vi "SensorColorSubVI.vi"(6 "Frecuencia in":bool, 7 "Frecuencia 1":bool=TRUE) -> (0 "Rojo":dbl format="%.2f", 1 "Azul":dbl, 2 "Verde":dbl format="%.2f", 3 "Sin Filtro":dbl format="%.2f")   [LabVIEW 2017]
uses:
  enumColor.ctl
  <vilib>/DAQmx/write.llb/DAQmx Write (Digital 1D Bool 1Chan 1Samp).vi
  <vilib>/DAQmx/read.llb/DAQmx Read (Counter DBL 1Chan 1Samp).vi
  <vilib>/DAQmx/create/channels.llb/DAQmx Create Channel (DO-Digital Output).vi
  <vilib>/DAQmx/create/channels.llb/DAQmx Create Channel (CI-Count Edges).vi
  <vilib>/DAQmx/miscellaneous.llb/DAQmx Fill In Error Info.vi
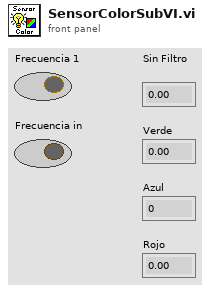
[diagram p1: front panel]
types:
  T1 = typedef "enumColor.ctl" = enum16{"Inicio", "SinFiltro1", "SinFiltro2", "SinFiltro3", "Rojo1", "Rojo2", "Rojo3", "Verde1", "Verde2", "Verde3", "Azul1", "Azul2", "Azul3", "Cierre"}
  T2 = cluster{"task out":refnum<k21>, "error out":errorcluster}
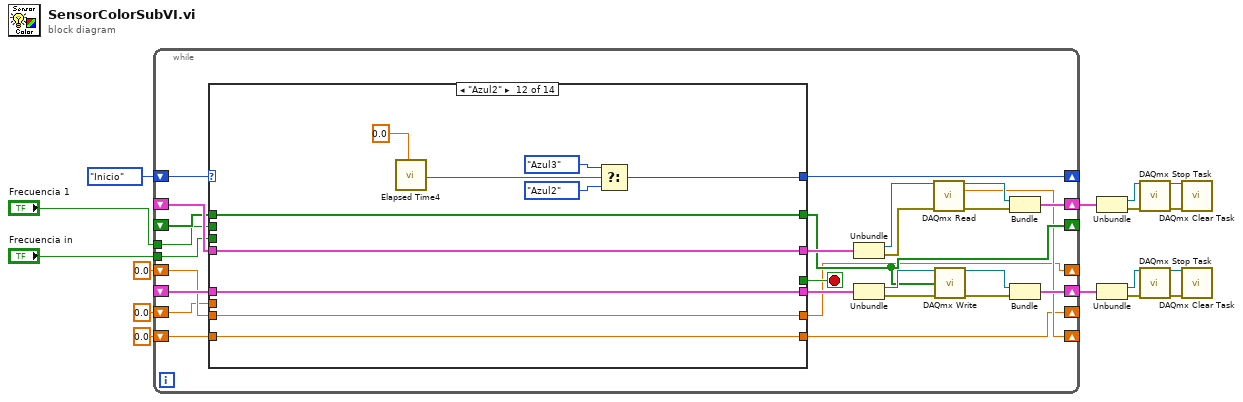
[diagram p0: block diagram]
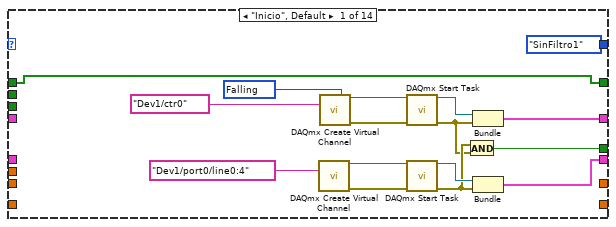
[diagram p2: hidden frame]
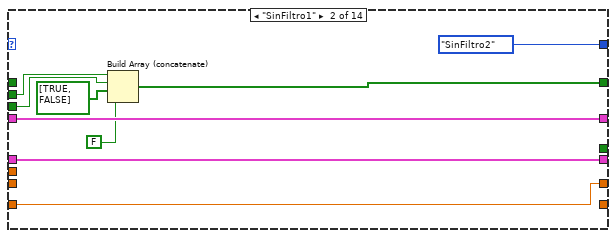
[diagram p3: hidden frame]
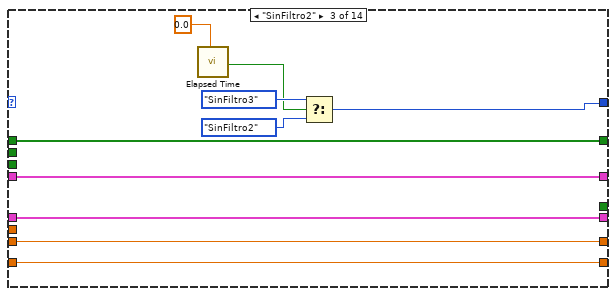
[diagram p4: hidden frame]
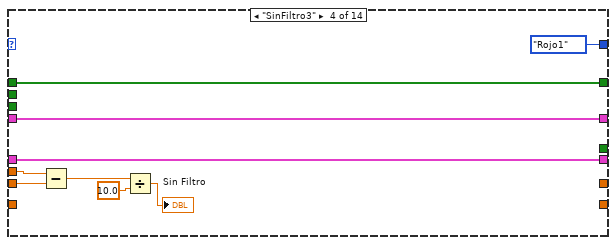
[diagram p5: hidden frame]
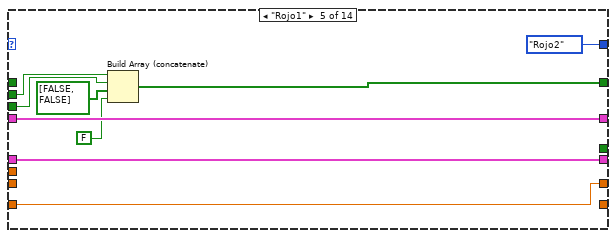
[diagram p6: hidden frame]
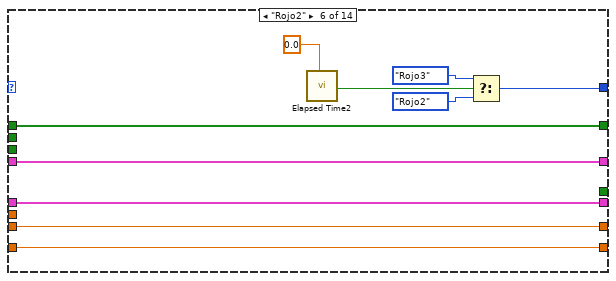
[diagram p7: hidden frame]
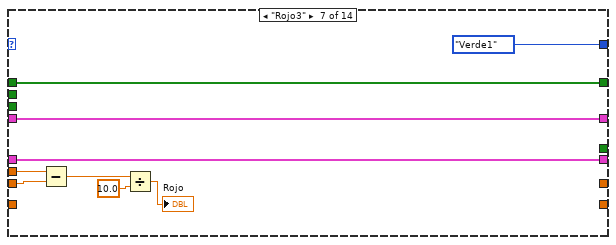
[diagram p8: hidden frame]
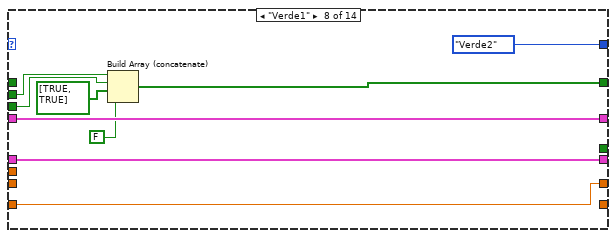
[diagram p9: hidden frame]
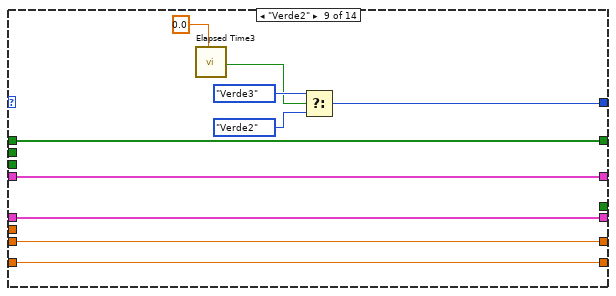
[diagram p10: hidden frame]
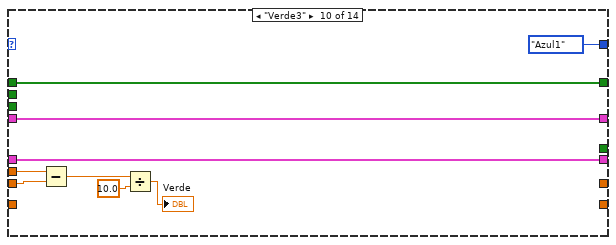
[diagram p11: hidden frame]
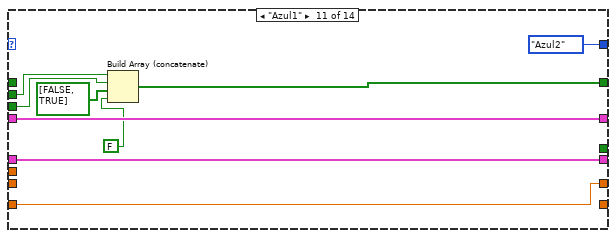
[diagram p12: hidden frame]
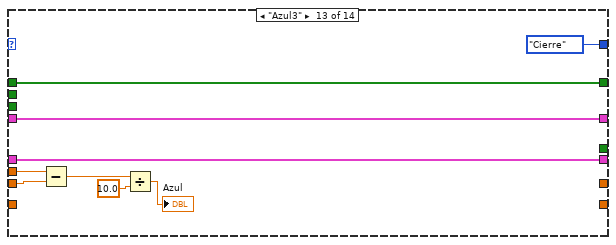
[diagram p13: hidden frame]
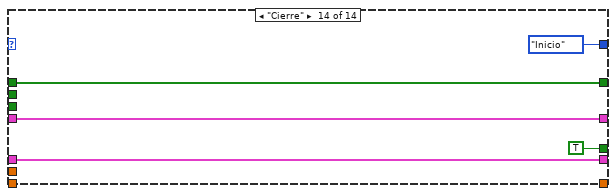
[diagram p14: hidden frame]
diagram:
  n1 = while {
    shift-right: [w42] -> _
    shift-left: enumColor."Inicio" -> [w27]
    shift-right: [w28] -> w14
    shift-left: _ -> [w29]
    shift-right: [w36] -> w13
    shift-left: _ -> [w33]
    tunnel: "Frecuencia 1" -> [w17]
    tunnel: "Frecuencia in" -> [w18]
    shift-right: [w26] -> _
    shift-left: _ -> [w25]
    shift-right: [w24] -> _
    shift-left: 0.0 ("data") -> [w23]
    shift-right: [w22] -> _
    shift-left: 0.0 ("data") -> [w21]
    shift-right: [w20] -> _
    shift-left: 0.0 ("data") -> [w19]
    stop <- w43 stop-if-true
    n2 = case shown="\"Azul2\"" w27 {
      tunnel: [w55 _ _ _ _ _ _ _ _ _ _ _ _ TRUE] -> w43
      tunnel: [w49 w68 w78 w87 w92 w106 w114 w119 w134 w142 w147 w162 w170 w175] -> w39
      tunnel: [enumColor."SinFiltro1" enumColor."SinFiltro2" w70 enumColor."Rojo1" enumColor."Rojo2" w102 enumColor."Verde1" enumColor."Verde2" w130 enumColor."Azul1" enumColor."Azul2" w158 enumColor."Cierre" enumColor."Inicio"] -> w42
      tunnel: w17 -> [_ w65 _ _ w95 _ _ w123 _ _ w151 _ _ _]
      tunnel: w18 -> [_ w64 _ _ w94 _ _ w122 _ _ w150 _ _ _]
      tunnel: [w46 w63 w77 w86 w93 w101 w113 w121 w129 w141 w149 w157 w169 w172] -> w26
      tunnel: w33 -> [_ w68 w78 w87 w92 w106 w114 w119 w134 w142 w147 w162 w170 w175]
      tunnel: [w47 w67 w76 w85 w91 w105 w115 w120 w133 w143 w148 w161 w171 w176] -> w30
      tunnel: w29 -> [_ w67 w76 w85 w91 w105 w115 w120 w133 w143 w148 w161 w171 w176]
      tunnel: w25 -> [w46 _ w77 w86 _ w101 w113 _ w129 w141 _ w157 w169 w172]
      tunnel: w23 -> [_ w61 w71 _ w89 w98 _ w117 w126 _ w146 w155 _ _]
      tunnel: [_ w61 w72 _ w89 w99 _ w117 w128 _ w146 w156 _ _] -> w22
      tunnel: w21 -> [_ _ w72 w80 _ w99 w112 _ w128 w139 _ w156 w165 _]
      tunnel: [_ _ w71 _ _ w98 _ _ w126 _ _ w155 _ _] -> w20
      tunnel: w19 -> [_ _ _ w81 _ _ w111 _ _ w140 _ _ w166 _]
      frame "Inicio", Default {
        w44 = 10171 items=["Rising"=10280, "Falling"=10171] ("edge")
        n3 = call-poly <vilib>:"DAQmx Create Virtual Channel.vi"("lines"=tag "Dev1/port0/line0:4") -> ("task out"=w59:refnum<k21>, "error out"=w58:errorcluster)  [unwired: 13 in]
        n4 = call-poly <vilib>:"DAQmx Create Virtual Channel.vi"("edge"=w44, "counter"=tag "Dev1/ctr0") -> ("task out"=w57:refnum<k21>, "error out"=w56:errorcluster)  [unwired: 12 in]
        n5 = call <vilib>:"DAQmx Start Task.vi"("task/channels in"=w57, "error in"=w56) -> ("task out"=w51:refnum<k21>, "error out"=w50:errorcluster)  [unwired: 12 in]
        n6 = call <vilib>:"DAQmx Start Task.vi"("task/channels in"=w59, "error in"=w58) -> ("task out"=w53:refnum<k21>, "error out"=w52:errorcluster)  [unwired: 12 in]
        n7 = And(x=w52, y=w50) -> (x .and. y?=w55:bool)
        n8 = Bundle("task out"=w51, "error out"=w50) -> (w49:T2)  [unwired: 1 in]
        n9 = Bundle("task out"=w53, "error out"=w52) -> (w47:T2)  [unwired: 1 in]
      }
      frame "SinFiltro1" {
        n10 = Build Array (concatenate)(w65, w64, bool[] [TRUE, FALSE], FALSE) -> (w63:bool[])
      }
      frame "SinFiltro2" {
        n11 = call "Elapsed Time"("Set Start Time (s)"=0.0) -> ("Time has Elapsed"=w73:bool)  [unwired: 11 in, 7 out]
        n12 = Select(t=enumColor."SinFiltro3", s=w73, f=enumColor."SinFiltro2") -> (s? t:f=w70:T1)
      }
      frame "SinFiltro3" {
        n13 = Subtract(x=w81, y=w80) -> (x-y=w84:dbl)
        n14 = Divide(x=w84, y=10.0) -> (x/y=→"Sin Filtro":dbl)
      }
      frame "Rojo1" {
        n15 = Build Array (concatenate)(w95, w94, bool[] [FALSE, FALSE], FALSE) -> (w93:bool[])
      }
      frame "Rojo2" {
        n16 = call "Elapsed Time2"("Set Start Time (s)"=0.0) -> ("Time has Elapsed"=w100:bool)  [unwired: 11 in, 7 out]
        n17 = Select(t=enumColor."Rojo3", s=w100, f=enumColor."Rojo2") -> (s? t:f=w102:T1)
      }
      frame "Rojo3" {
        n18 = Subtract(x=w111, y=w112) -> (x-y=w110:dbl)
        n19 = Divide(x=w110, y=10.0) -> (x/y=→"Rojo":dbl)
      }
      frame "Verde1" {
        n20 = Build Array (concatenate)(w123, w122, bool[] [TRUE, TRUE], FALSE) -> (w121:bool[])
      }
      frame "Verde2" {
        n21 = call "Elapsed Time3"("Set Start Time (s)"=0.0) -> ("Time has Elapsed"=w127:bool)  [unwired: 11 in, 7 out]
        n22 = Select(t=enumColor."Verde3", s=w127, f=enumColor."Verde2") -> (s? t:f=w130:T1)
      }
      frame "Verde3" {
        n23 = Subtract(x=w140, y=w139) -> (x-y=w137:dbl)
        n24 = Divide(x=w137, y=10.0 ("x")) -> (x/y=→"Verde":dbl)
      }
      frame "Azul1" {
        n25 = Build Array (concatenate)(w151, w150, bool[] [FALSE, TRUE], FALSE) -> (w149:bool[])
      }
      frame "Azul2" {
        n26 = call "Elapsed Time4"("Set Start Time (s)"=0.0) -> ("Time has Elapsed"=w154:bool)  [unwired: 11 in, 7 out]
        n27 = Select(t=enumColor."Azul3", s=w154, f=enumColor."Azul2") -> (s? t:f=w158:T1)
      }
      frame "Azul3" {
        n28 = Subtract(x=w166, y=w165) -> (x-y=w167:dbl)
        n29 = Divide(x=w167, y=10.0) -> (x/y=→"Azul":dbl)
      }
      frame "Cierre" {
      }
    }
    n30 = Unbundle(w39) -> ("task out"=w38:refnum<k21>, "error out"=w37:errorcluster)
    n31 = Unbundle(w30) -> ("task out"=w41:refnum<k21>, "error out"=w40:errorcluster)
    n32 = call-poly <vilib>:"DAQmx Read.vi"("task/channels in"=w38, "error in"=w37) -> ("task out"=w35:refnum<k21>, "data"=w24:dbl, "error out"=w34:errorcluster)  [unwired: 11 in]
    n33 = call-poly <vilib>:"DAQmx Write.vi"("task/channels in"=w41, "data"=w26, "error in"=w40) -> ("task out"=w32:refnum<k21>, "error out"=w31:errorcluster)  [unwired: 10 in, 1 out]
    n34 = Bundle("task out"=w35, "error out"=w34) -> (w36:T2)  [unwired: 1 in]
    n35 = Bundle("task out"=w32, "error out"=w31) -> (w28:T2)  [unwired: 1 in]
  }
  n36 = Unbundle(w13) -> ("task out"=w10:refnum<k21>, "error out"=w9:errorcluster)
  n37 = Unbundle(w14) -> ("task out"=w12:refnum<k21>, "error out"=w11:errorcluster)
  n38 = call <vilib>:"DAQmx Stop Task.vi"("task/channels in"=w10, "error in"=w9) -> ("task out"=w6:refnum<k21>, "error out"=w5:errorcluster)  [unwired: 12 in]
  n39 = call <vilib>:"DAQmx Stop Task.vi"("task/channels in"=w12, "error in"=w11) -> ("task out"=w8:refnum<k21>, "error out"=w7:errorcluster)  [unwired: 12 in]
  n40 = call <vilib>:"DAQmx Clear Task.vi"("task in"=w6, "error in"=w5) -> ()  [unwired: 13 in, 1 out]
  n41 = call <vilib>:"DAQmx Clear Task.vi"("task in"=w8, "error in"=w7) -> ()  [unwired: 13 in, 1 out]
